vi "Configure Frequency.vi"(0 "VISA resource name":refnum<visa-resource-name>, 1 "Reference Frequency (0 Hz)":dbl, 2 "Enable Reference Frequency (F:Disable)":bool, 5 "Frequency (100 kHz)":dbl=100000.0, 7 "Offset Frequency (0 Hz)":dbl, 9 "Frequency Multiplier (1.0)":dbl=1.0, 11 "error in (no error)":errorcluster, 12 "Phase Adjustment (0 rad)":dbl, 13 "Phase Noise Offsets (1: Below 10 kHz)":u16(ring)=1 items=["Below 10 kHz"=1, "Above 10 kHz"=2]) -> (4 "VISA resource name out":refnum<visa-resource-name>, 15 "error out":errorcluster)   [LabVIEW 2012, in "Agilent PSG MXG Series.lvlib"]
doc: "Configures frequency mode, frequency channel, frequency multiplier and PLL bandwidth."
uses:
  <instrlib>/Agilent PSG MXG Series/Agilent PSG MXG Series.lvlib
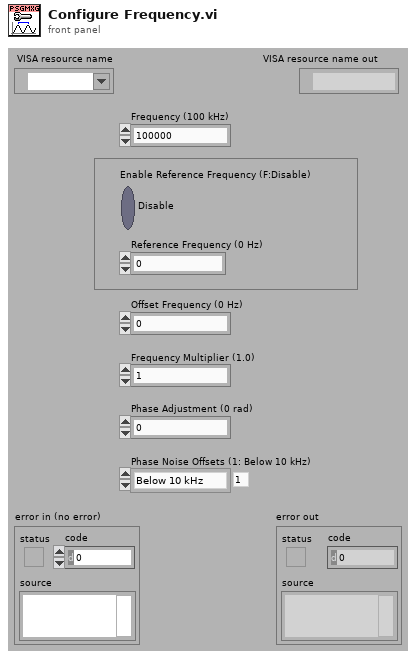
[diagram p1: front panel]
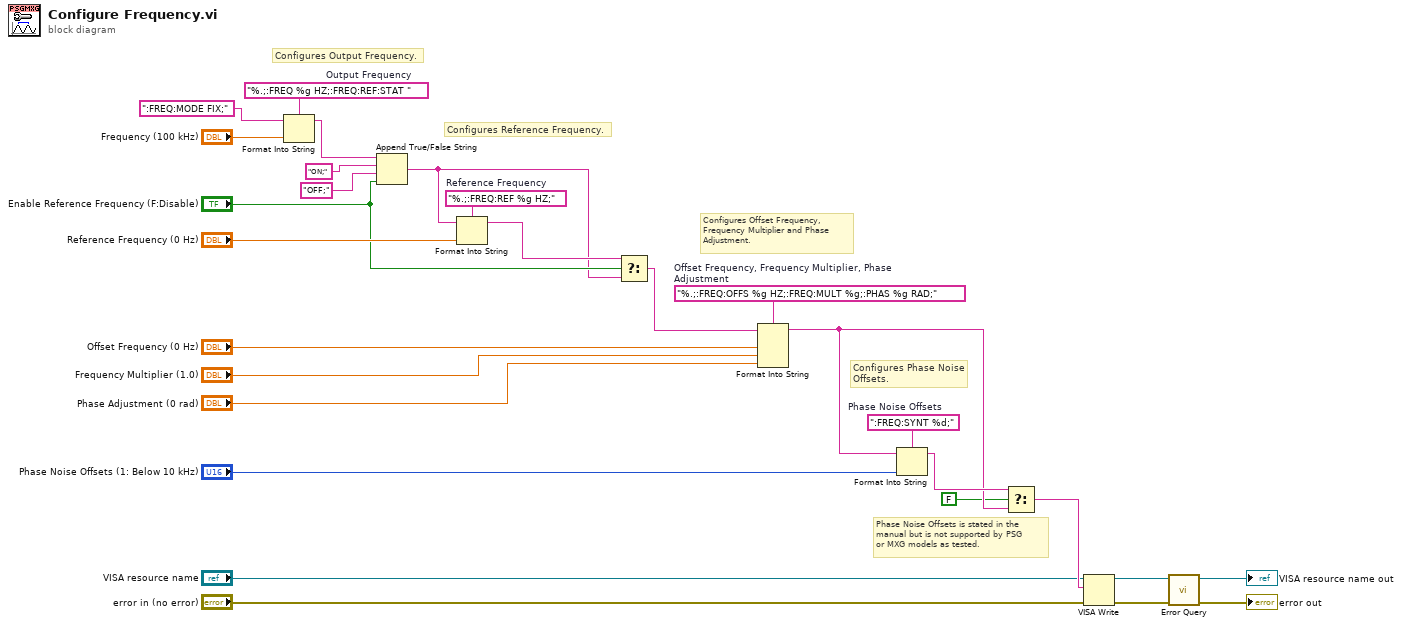
[diagram p0: block diagram]
diagram:
  w15 = "%.;:FREQ:REF %g HZ;"  # Reference Frequency
  w19 = "%.;:FREQ:OFFS %g HZ;:FREQ:MULT %g;:PHAS %g RAD;"  # Offset Frequency, Frequency Multiplier, Phase Adjustment
  w24 = "%.;:FREQ %g HZ;:FREQ:REF:STAT "  # Output Frequency
  w26 = ":FREQ:SYNT %d;"  # Phase Noise Offsets
  # "Phase Noise Offsets is stated in the\nmanual but is not supported by PSG\nor MXG models as tested."
  # "Configures Reference Frequency."
  # "Configures Output Frequency."
  # "Configures Phase Noise\nOffsets."
  # "Configures Offset Frequency,\nFrequency Multiplier and Phase\nAdjustment."
  n1 = Format Into String(format string=w24, initial string=":FREQ:MODE FIX;", "Frequency (100 kHz)") -> (resulting string=w22:string)  [unwired: 1 in, 1 out]
  n2 = Append True/False String(1:"Enable Reference Frequency (F:Disable)", 2:"OFF;" ("false string"), 3:"ON;" ("false string"), 4:w22) -> (0:w11:string)
  n3 = Format Into String(format string=w15, initial string=w11, "Reference Frequency (0 Hz)") -> (resulting string=w12:string)  [unwired: 1 in, 1 out]
  n4 = Select(t=w12, s="Enable Reference Frequency (F:Disable)", f=w11) -> (s? t:f=w10:string)
  n5 = Format Into String(format string=w19, initial string=w10, "Offset Frequency (0 Hz)", "Frequency Multiplier (1.0)", "Phase Adjustment (0 rad)") -> (resulting string=w8:string)  [unwired: 1 in, 1 out]
  n6 = Format Into String(format string=w26, initial string=w8, "Phase Noise Offsets (1: Below 10 kHz)") -> (resulting string=w9:string)  [unwired: 1 in, 1 out]
  n7 = Select(t=w9, s=FALSE, f=w8) -> (s? t:f=w25:string)
  n8 = VISA Write(VISA resource name="VISA resource name", write buffer=w25, error in (no error)="error in (no error)") -> (VISA resource name out=w28:refnum<visa-resource-name>, error out=w27:errorcluster)  [unwired: 1 out]
  n9 = call <instrlib>:"Error Query.vi"("error in (no error)"=w27, "VISA resource name"=w28) -> ("error out"=→"error out":errorcluster, "VISA resource name out"=→"VISA resource name out":refnum<visa-resource-name>)  [unwired: 8 out]
